vi "Handle.vi"(11 "Base Queue in":refnum<class "Base Queue.lvclass">) -> (2 "Destroy?":bool, 3 "Base Queue out":refnum<class "Base Queue.lvclass">)   [LabVIEW 2021, in "jettl.lvlib" / "Base Queue.lvlib" / "Base Queue.lvclass"]
uses:
  Base Queue.lvclass
  C:/git/jettl/src/jettl/Queue/Queue.lvclass
  State/Error State/Error State.lvclass
  C:/git/jettl/src/jettl/Base Queue/State/State/State.lvclass
  Base Queue.lvclass/Base Queue.ctl
  State/State/State.lvclass
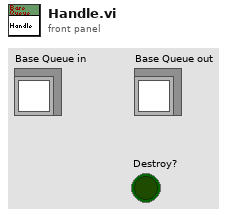
[diagram p1: front panel]
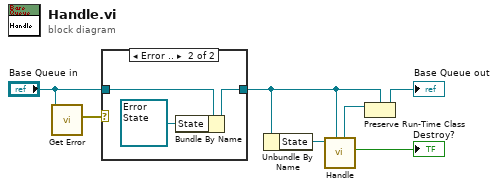
[diagram p0: block diagram]
diagram:
  n1 = call-dynamic "Get Error.vi"("Base Queue in"="Base Queue in") -> ("Error"=w3:errorcluster)  [unwired: 10 in]
  n2 = case shown="Error .." w3 {
    tunnel: [w8 w10] -> w1
    tunnel: "Base Queue in" -> [w8 w11]
    frame No Error {
    }
    frame Error {
      n3 = Bundle By Name(cluster=w11, "State"=refnum<class "Error State.lvclass"> refnum ("jettl.lvlib:jettl Queue Actor.lvlib:Error State.lvclass")) -> (w10:refnum<class "Base Queue.lvclass">)
    }
  }
  n4 = Unbundle By Name(w1) -> ("State"=w7:refnum<class "State.lvclass">)
  n5 = call-dynamic "Handle.vi"("Queue in"=w1, "State in"=w7) -> ("Destroy?"=→"Destroy?":bool, "Queue out"=w6:refnum<class "Queue.lvclass">)  [unwired: 8 in]
  n6 = Preserve Run-Time Class(object in=w6, 2:w1) -> (object out=→"Base Queue out":refnum<class "Base Queue.lvclass">)  [unwired: 1 in, 1 out]
